vi "Custom Classification.vi"() -> ()   [LabVIEW 2016]
uses:
  <vilib>/vision/Classification.llb/IMAQ Classifier Nearest Neighbor Training Results.ctl
  <vilib>/vision/NI_Vision_Development_Module.lvlib
panel:
  out "Sample2":T1(plugin-control)
  out "Sample1":T1(plugin-control)
  out "Training Results":T2[](array[typedef]) {"Standard Deviation" format="%.6f"}
  out "FVector2":dbl[](array[numeric])
  out "FVector1":dbl[](array[numeric])
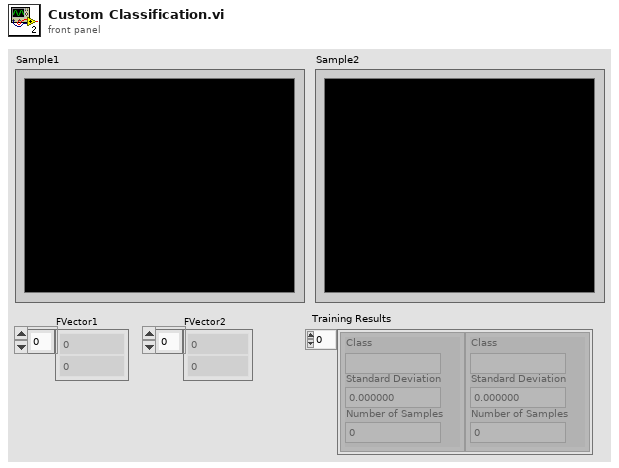
[diagram p1: front panel]
types:
  T1 = typedef "IMAQ Image.ctl" = refnum<image>
  T2 = typedef "IMAQ Classifier Nearest Neighbor Training Results.ctl" = cluster{"Class":string, "Standard Deviation":sgl, "Number of Samples":i32}
  T3 = typedef "Particle Parameters" = i32
  T4 = typedef "IMAQ Classifier Session.ctl" = refnum<k1>
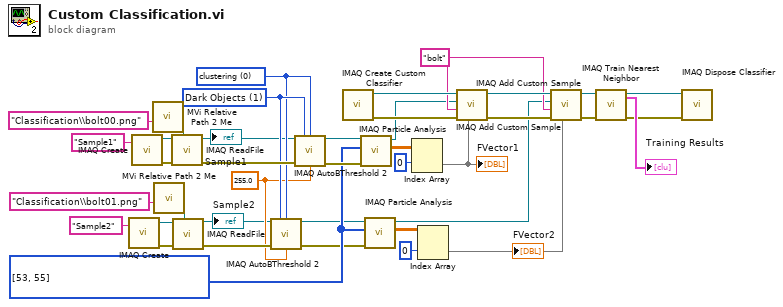
[diagram p0: block diagram]
diagram:
  w15 = sgl 255.0 ("Replace Value (1)")
  w22 = T3[] [53, 55] items=["Center of Mass X", "Center of Mass Y", "First Pixel X", "First Pixel Y", "Bounding Rect Left", "Bounding Rect Top", "Bounding Rect Right", "Bounding Rect Bottom", "Max Feret Diameter Start X", "Max Feret Diameter Start Y", "Max Feret Diameter End X", "Max Feret Diameter End Y", "Max Horiz. Segment Length Left", "Max Horiz. Segment Length Right", "Max Horiz. Segment Length Row", "-", "Bounding Rect Width", "Bounding Rect Height", "Bounding Rect Diagonal", "Perimeter", "Convex Hull Perimeter", "Holes' Perimeter", "Max Feret Diameter", "Equivalent Ellipse Major Axis", "Equivalent Ellipse Minor Axis", "Equivalent Ellipse Minor Axis (Feret)", "Equivalent Rect Long Side", "Equivalent Rect Short Side", "Equivalent Rect Diagonal", "Equivalent Rect Short Side (Feret)", "Average Horiz. Segment Length", "Average Vert. Segment Length", "Hydraulic Radius", "Waddel Disk Diameter", "-", "Area", "Holes' Area", "Particle & Holes' Area", "Convex Hull Area", "Image Area", "-", "Number of Holes", "Number of Horiz. Segments", "Number of Vert. Segments", "-", "Orientation", "Max Feret Diameter Orientation", "-", "% Area/Image Area", "% Area/(Particle & Holes' Area)", "Ratio of Equivalent Ellipse Axes", "Ratio of Equivalent Rect Sides", "-", "Elongation Factor", "Compactness Factor", "Heywood Circularity Factor", "Type Factor", "-", "Sum X", "Sum Y", "Sum XX", "Sum XY", "Sum YY", "Sum XXX", "Sum XXY", "Sum XYY", "Sum YYY", "-", "Moment of Inertia XX", "Moment of Inertia XY", "Moment of Inertia YY", "Moment of Inertia XXX", "Moment of Inertia XXY", "Moment of Inertia XYY", "Moment of Inertia YYY", "Norm. Moment of Inertia XX", "Norm. Moment of Inertia XY", "Norm. Moment of Inertia YY", "Norm. Moment of Inertia XXX", "Norm. Moment of Inertia XXY", "Norm. Moment of Inertia XYY", "Norm. Moment of Inertia YYY", "Hu Moment 1", "Hu Moment 2", "Hu Moment 3", "Hu Moment 4", "Hu Moment 5", "Hu Moment 6", "Hu Moment 7"] ("Pixel Measurements")
  w24 = 0 items=["clustering", "entropy", "metric", "moments", "inter-class variance"] ("Method (clustering)")
  w25 = u32 1 items=["Bright Objects", "Dark Objects"] ("Look For (Bright Objects)")
  w28 = "bolt" ("Class")
  n1 = call "IMAQ Create"("Image Name"="Sample2") -> ("Src"=w30:T1, "error out"=w31:errorcluster)  [unwired: 4 in]
  n2 = call "IMAQ Create"("Image Name"="Sample1") -> ("Src"=w34:T1, "error out"=w35:errorcluster)  [unwired: 4 in]
  n3 = call "MVi Relative Path 2 Me.vi"("Relative Path"="Classification\\bolt00.png") -> ("Appended Dir"=w5:path)  [unwired: 5 in, 1 out]
  n4 = call "MVi Relative Path 2 Me.vi"("Relative Path"="Classification\\bolt01.png") -> ("Appended Dir"=w3:path)  [unwired: 5 in, 1 out]
  n5 = call "IMAQ ReadFile"("File Path"=w5, "error in (no error)"=w35, "Image"=w34) -> ("error out"=w27:errorcluster, "Image Out"=w7:T1)  [unwired: 4 in, 3 out]
  "Sample1" <- w7
  n6 = call "IMAQ ReadFile"("File Path"=w3, "error in (no error)"=w31, "Image"=w30) -> ("error out"=w26:errorcluster, "Image Out"=w8:T1)  [unwired: 4 in, 3 out]
  "Sample2" <- w8
  n7 = call "IMAQ AutoBThreshold 2"("Image Src"=w8, "Look For (Bright Objects)"=w25, "Method (clustering)"=w24, "error in (no error)"=w26, "Replace Value (1)"=w15) -> ("Image Dst Out"=w9:T1, "error out"=w21:errorcluster)  [unwired: 8 in, 1 out]
  n8 = call "IMAQ AutoBThreshold 2"("Image Src"=w7, "Look For (Bright Objects)"=w25, "Method (clustering)"=w24, "error in (no error)"=w27, "Replace Value (1)"=w15) -> ("Image Dst Out"=w10:T1, "error out"=w23:errorcluster)  [unwired: 8 in, 1 out]
  n9 = call "IMAQ Create Custom Classifier"() -> ("error out"=w39:errorcluster, "Classifier Session"=w40:T4)  [unwired: 10 in]
  n10 = call "IMAQ Particle Analysis"("error in (no error)"=w23, "Pixel Measurements"=w22, "Image"=w10) -> ("Particle Measurements (Pixels)"=w20:dbl[][], "Image Out (duplicate)"=w17:T1)  [unwired: 3 in, 4 out]
  n11 = call "IMAQ Particle Analysis"("error in (no error)"=w21, "Pixel Measurements"=w22, "Image"=w9) -> ("Particle Measurements (Pixels)"=w18:dbl[][], "Image Out (duplicate)"=w16:T1)  [unwired: 3 in, 4 out]
  n12 = Index Array(array=w20, index (row)=0 ("disabled index (col)")) -> (element=w19:dbl[])  [unwired: 1 in]
  "FVector1" <- w19
  n13 = Index Array(array=w18, index (row)=0 ("disabled index (col)")) -> (element=w14:dbl[])  [unwired: 1 in]
  "FVector2" <- w14
  n14 = call "IMAQ Add Custom Sample"("Feature Vector"=w19, "error in (no error)"=w39, "Class"=w28, "Image"=w17, "Classifier Session"=w40) -> ("error out"=w38:errorcluster, "Classifier Session (dup)"=w29:T4)  [unwired: 5 in]
  n15 = call "IMAQ Add Custom Sample"("Feature Vector"=w14, "error in (no error)"=w38, "Class"=w28, "Image"=w16, "Classifier Session"=w29) -> ("error out"=w36:errorcluster, "Classifier Session (dup)"=w37:T4)  [unwired: 5 in]
  n16 = call "IMAQ Train Nearest Neighbor"("error in (no error)"=w36, "Classifier Session"=w37) -> ("error out"=w1:errorcluster, "Classifier Session (dup)"=w2:T4, "Training Results"=→"Training Results":T2[])  [unwired: 6 in, 1 out]
  n17 = call "IMAQ Dispose Classifier"("error in (no error)"=w1, "Classifier Session"=w2) -> ()  [unwired: 9 in, 1 out]
